vi "AAL Resample (const to Variable, complex single-channel).vi"(7 "reset? (True)":bool=TRUE, 8 "error in (no error)":errorcluster, 9 "config":T1={"timing jitter"=enum."Interpolation", "anti-aliasing?"=TRUE, "filter prototype"={"coefficients"=[], "factor"=1}} {"filter prototype"."coefficients" format="%.2f"}, 10 "time":dbl[](array[numeric]) format="%.2f", 11 "X":cdb[](array[numeric])) -> (0 "error out":errorcluster, 1 "offset":i32, 2 "time stamps":dbl[](array[numeric]) format="%.2f", 3 "Y":cdb[](array[numeric]) format="%.2f")   [LabVIEW 2010, in "NI_AALPro.lvlib"]
doc: "Perform an arbitrary resampling on the input signal."
uses:
  NI_AALPro.lvlib
  lvanlys.dll
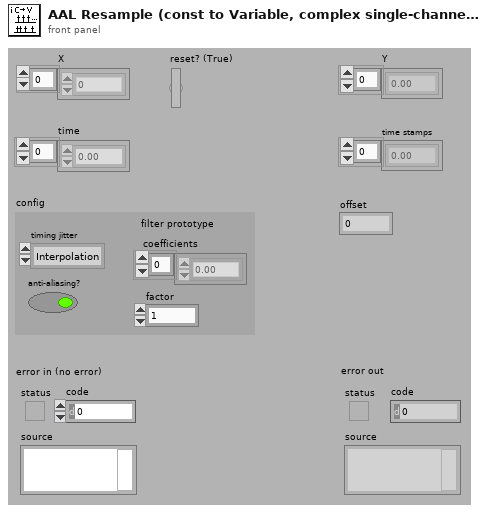
[diagram p1: front panel]
types:
  T1 = cluster{"timing jitter":enum32{"Interpolation", "Rounding"}, "anti-aliasing?":bool, "filter prototype":cluster{"coefficients":dbl[], "factor":i32}}
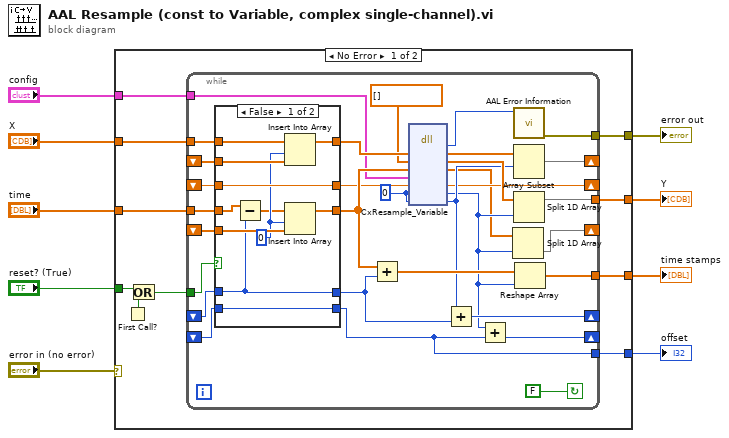
[diagram p0: block diagram]
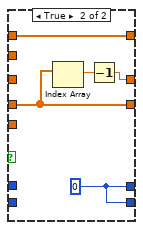
[diagram p2: hidden frame]
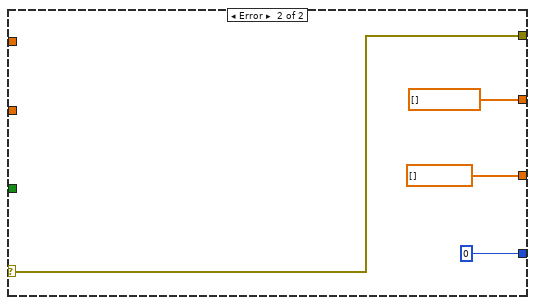
[diagram p3: hidden frame]
diagram:
  n1 = case shown="No Error" "error in (no error)" {
    selector: "error in (no error)" -> [_ w71]
    tunnel: "config" -> [w18 _]
    tunnel: "reset? (True)" -> [w17 _]
    tunnel: "time" -> [w11 _]
    tunnel: [w15 dbl[] []] -> w6
    tunnel: [w14 cdb[] []] -> w5
    tunnel: [w13 0] -> w4
    tunnel: [w12 w71] -> w3
    tunnel: "X" -> [w10 _]
    frame No Error {
      n2 = First Call?() -> (First Call?: T/F=w19:bool)
      n3 = Or(x=w17, y=w19) -> (x .or. y?=w16:bool)
      n4 = while {
        tunnel: [w43] -> w14
        tunnel: [w34] -> w15
        shift-right: [w25] -> _
        shift-left: _ -> [w45]
        shift-right: [w51] -> _
        shift-left: _ -> [w46]
        tunnel: w10 -> [w49]
        tunnel: w11 -> [w47]
        shift-right: [w28] -> _
        shift-left: _ -> [w44]
        tunnel: w16 -> [w22]
        tunnel: w18 -> [w26]
        shift-right: [w42] -> _
        shift-left: _ -> [w21]
        tunnel: [w38] -> w13
        shift-right: [w37] -> _
        shift-left: _ -> [w39]
        tunnel: [w35] -> w12
        stop <- FALSE continue-if-true
        w32 = 0
        n5 = case shown="False" w22 {
          tunnel: [w61 w67] -> w48
          tunnel: w49 -> [w59 w67]
          tunnel: [w56 w66] -> w33
          tunnel: w47 -> [w55 w66]
          tunnel: [w62 w64] -> w27
          tunnel: w46 -> [w58 _]
          tunnel: w45 -> [w60 _]
          tunnel: w44 -> [w62 _]
          tunnel: w21 -> [w53 _]
          tunnel: [w53 w63] -> w20
          tunnel: w39 -> [w52 _]
          tunnel: [w52 w63] -> w38
          frame False {
            w57 = 0 ("Index")
            n6 = Subtract(x=w55, y=w53) -> (x-y=w54:dbl[])
            n7 = Insert Into Array(array=w59, index=w57, new element=w58) -> (w61:cdb[])
            n8 = Insert Into Array(array=w54, index=w57, new element=w60) -> (w56:dbl[])
          }
          frame True {
            w63 = 0
            n9 = Index Array(array=w66) -> (element=w65:dbl)  [unwired: 1 in]
            n10 = Decrement(x=w65) -> (x-1=w64:dbl)
          }
        }
        n11 = Add(x=w33, y=w20) -> (x+y=w41:dbl[])
        n12 = dll-call lib="C:/Program Files/National Instruments/LabVIEW 2010/resource/lvanlys.*" fn="CxResample_Variable"("X"=w48, "X"=cdb[] [], "timeH"=w33, "config"=w26, "last_sample_time"=w27, "out_len"=w32, "xLeftOverIdx"=w32) -> (w36:i32, "X"=w40:cdb[], "X"=w31:cdb[], "timeH"=w23:dbl[], "last_sample_time"=w28:dbl, "out_len"=w24:i32, "xLeftOverIdx"=w29:i32)  [unwired: 4 in, 2 out]
        n13 = Add(x=w29, y=w20) -> (x+y=w42:i32)
        n14 = Add(x=w24, y=w38) -> (x+y=w37:i32)
        n15 = Split 1D Array(array=w23, index=w24) -> (second subarray=w25:dbl[])  [unwired: 1 out]
        n16 = call "AAL Error Information.vi"("error code"=w36) -> ("error out"=w35:errorcluster)  [unwired: 10 in]
        n17 = Array Subset(array=w40, index=w29) -> (w51:cdb[])  [unwired: 1 in]
        n18 = Split 1D Array(array=w31, index=w24) -> (first subarray=w43:cdb[])  [unwired: 1 out]
        n19 = Reshape Array(w41, w24) -> (w34:dbl[])
      }
    }
    frame Error {
    }
  }
  "time stamps" <- w6
  "Y" <- w5
  "offset" <- w4
  "error out" <- w3
